vi "MultColLB-pair Operations.vi"() -> ()   [LabVIEW 2020, in "MulColLBTable-pair.lvclass"]
uses:
  MulColLBTable-pair.lvclass
  MulColLBTable/MulColLBTable.lvclass
panel:
  in  "Multicol-pair OBJ":refnum<class "MulColLBTable-pair.lvclass">
  out "Multicol-pair":refnum<class "MulColLBTable-pair.lvclass">
  in  "Lisbox Ref 2":refnum<vi>
  in  "Listbox Ref 1":refnum<vi>
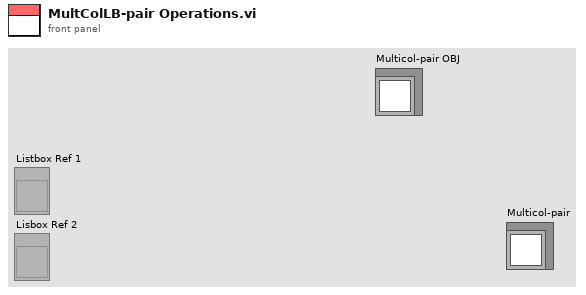
[diagram p1: front panel]
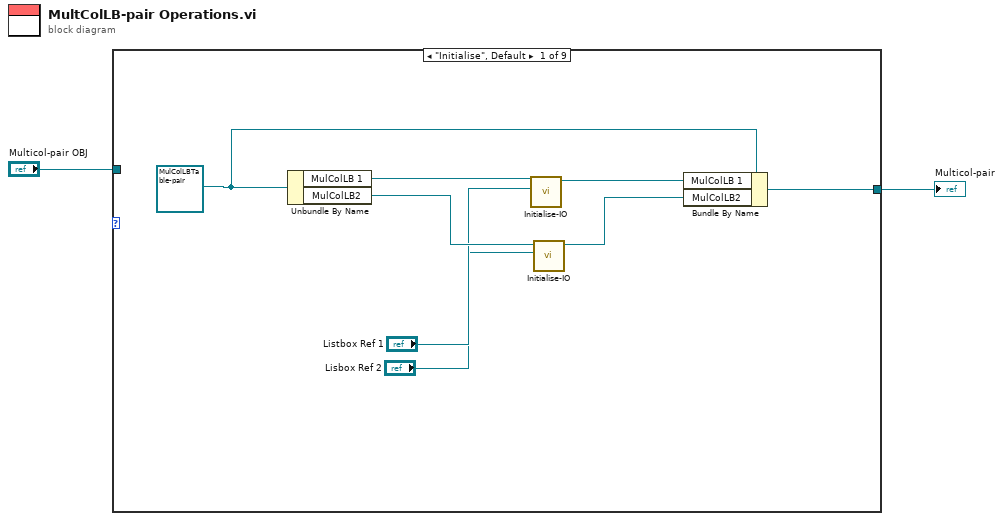
[diagram p0: block diagram]
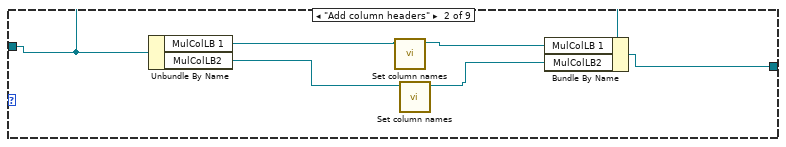
[diagram p2: hidden frame]
diagram:
  n1 = case shown="\"Initialise\", Default" w3 {
    tunnel: [w4 w13 _ _ _ _ _ _ _] -> w2
    tunnel: "Multicol-pair OBJ" -> [_ w12 _ _ _ _ _ _ _]
    frame "Initialise", Default {
      w7 = refnum<class "MulColLBTable-pair.lvclass"> refnum ("MulColLBTable-pair.lvclass")
      n2 = Unbundle By Name(w7) -> ("MulColLB 1"=w11:refnum<class "MulColLBTable.lvclass">, "MulColLB2"=w10:refnum<class "MulColLBTable.lvclass">)
      n3 = call "Initialise-IO.vi"("Multicolumn Listbox"="Listbox Ref 1", "MulColLBTable.lvclass"=w11) -> ("MulColLBTable.lvclass out"=w6:refnum<class "MulColLBTable.lvclass">)  [unwired: 8 in, 1 out]
      n4 = call "Initialise-IO.vi"("Multicolumn Listbox"="Lisbox Ref 2", "MulColLBTable.lvclass"=w10) -> ("MulColLBTable.lvclass out"=w5:refnum<class "MulColLBTable.lvclass">)  [unwired: 8 in, 1 out]
      n5 = Bundle By Name(cluster=w7, "MulColLB 1"=w6, "MulColLB2"=w5) -> (w4:refnum<class "MulColLBTable-pair.lvclass">)
    }
    frame "Add column headers" {
      n6 = Unbundle By Name(w12) -> ("MulColLB 1"=w17:refnum<class "MulColLBTable.lvclass">, "MulColLB2"=w15:refnum<class "MulColLBTable.lvclass">)
      n7 = call "Set column names.vi"("MulColLBTable.lvclass"=w17) -> ("MulColLBTable.lvclass 2"=w16:refnum<class "MulColLBTable.lvclass">)  [unwired: 9 in, 1 out]
      n8 = call "Set column names.vi"("MulColLBTable.lvclass"=w15) -> ("MulColLBTable.lvclass 2"=w14:refnum<class "MulColLBTable.lvclass">)  [unwired: 9 in, 1 out]
      n9 = Bundle By Name(cluster=w12, "MulColLB 1"=w16, "MulColLB2"=w14) -> (w13:refnum<class "MulColLBTable-pair.lvclass">)
    }
    frame "Add rows - bulk" {
    }
    frame "Stack row - single" {
    }
    frame "Stack row - multi" {
    }
    frame "Select row" {
    }
    frame "Delete row - single" {
    }
    frame "Delete row - multi" {
    }
    frame "Destroy" {
    }
  }
  "Multicol-pair" <- w2
